vi "gRPC Status to Node Status.vi"(2 "gRPC Status":T1) -> (4 "Node Status":T10 {"Monitor Doubles"."4" format="%#_9g"; "Monitor Doubles"."3" format="%#_9g"; "Monitor Doubles"."2" format="%#_9g"; "Monitor Doubles"."1" format="%#_9g"})   [LabVIEW 2021, in "CIFCorePluginWrapper.lvlib"]
uses:
  Common/Typedef/gRPC Reported Plugin Status.ctl
  Common/Typedef/Plugin State.ctl
  Common/Typedef/Timing Statistics.ctl
  Common/Typedef/Timing Stats Base.ctl
  Common/Typedef/FIFO Statistics.ctl
  Common/Typedef/Simple Error.ctl
  Common/Typedef/Monitor Doubles.ctl
  Common/Typedef/Monitor U64.ctl
  Common/Typedef/Monitor I64.ctl
  CIFCorePlugin_client/RPC Messages/cif_plugincore_StatusData.ctl
  CIFCorePlugin_client/RPC Messages/cif_plugincore_StatusData_State.ctl
  CIFCorePlugin_client/RPC Messages/cif_plugincore_TimingStatistics.ctl
  CIFCorePlugin_client/RPC Messages/cif_plugincore_TimingStatsBasic.ctl
  CIFCorePlugin_client/RPC Messages/cif_plugincore_FifoStatistics.ctl
  CIFCorePlugin_client/RPC Messages/cif_plugincore_Error.ctl
  CIFCorePlugin_client/RPC Messages/cif_plugincore_MonitorDoubles.ctl
  CIFCorePlugin_client/RPC Messages/cif_plugincore_MonitorU64.ctl
  CIFCorePlugin_client/RPC Messages/cif_plugincore_MonitorI64.ctl
  CIFCorePluginWrapper.lvlib
  Common/CIFCoreCommon.lvlib
  CIFCorePlugin_client/CIFCorePlugin_client.lvlib
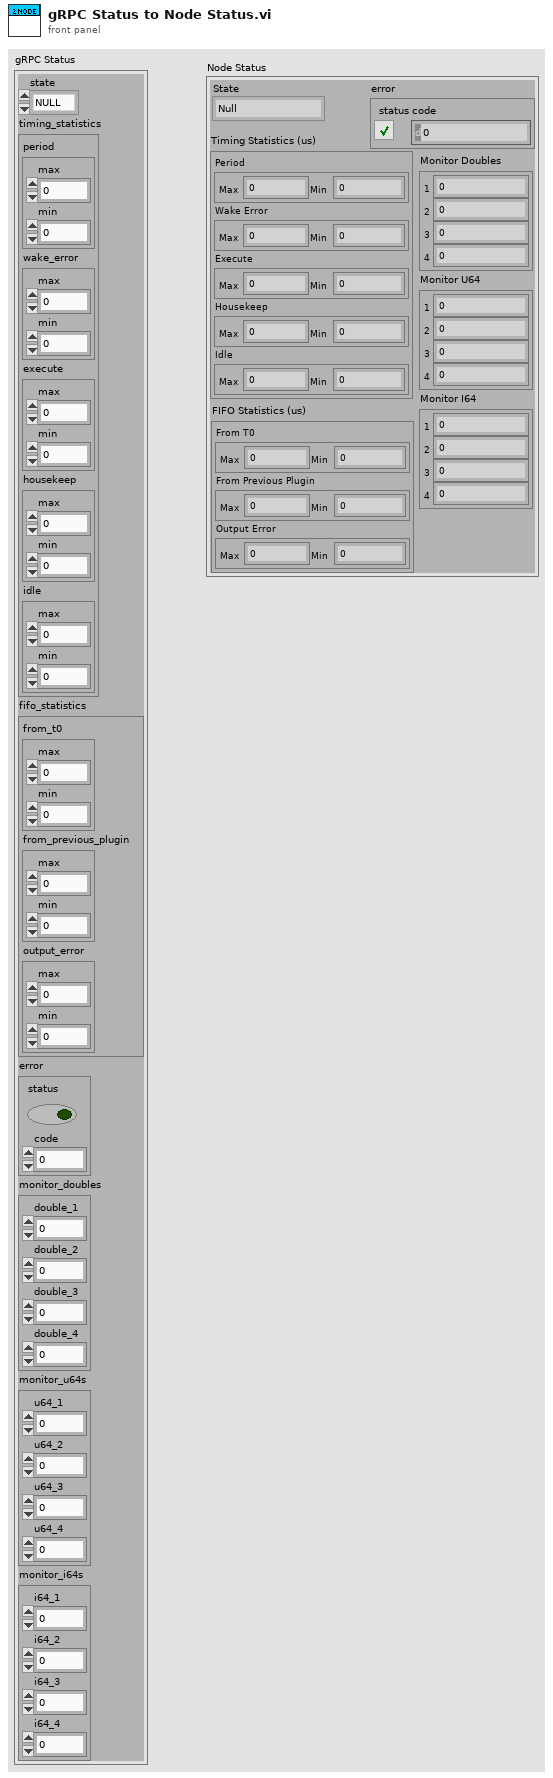
[diagram p1: front panel]
types:
  T1 = typedef "CIFCorePlugin_client.lvlib/cif_plugincore_StatusData.ctl" = cluster{"state":T2, "timing_statistics":T3, "fifo_statistics":T5, "error":T6, "monitor_doubles":T7, "monitor_u64s":T8, "monitor_i64s":T9}
  T2 = typedef "CIFCorePlugin_client.lvlib/cif_plugincore_StatusData_State.ctl" = enum32{"NULL", "CREATING", "LISTENING", "RUNNING", "CLEANINGUP", "DESTROYING"}
  T3 = typedef "CIFCorePlugin_client.lvlib/cif_plugincore_TimingStatistics.ctl" = cluster{"period":T4, "wake_error":T4, "execute":T4, "housekeep":T4, "idle":T4}
  T4 = typedef "CIFCorePlugin_client.lvlib/cif_plugincore_TimingStatsBasic.ctl" = cluster{"max":i32, "min":i32}
  T5 = typedef "CIFCorePlugin_client.lvlib/cif_plugincore_FifoStatistics.ctl" = cluster{"from_t0":T4, "from_previous_plugin":T4, "output_error":T4}
  T6 = typedef "CIFCorePlugin_client.lvlib/cif_plugincore_Error.ctl" = cluster{"status":bool, "code":i32}
  T7 = typedef "CIFCorePlugin_client.lvlib/cif_plugincore_MonitorDoubles.ctl" = cluster{"double_1":dbl, "double_2":dbl, "double_3":dbl, "double_4":dbl}
  T8 = typedef "CIFCorePlugin_client.lvlib/cif_plugincore_MonitorU64.ctl" = cluster{"u64_1":u64, "u64_2":u64, "u64_3":u64, "u64_4":u64}
  T9 = typedef "CIFCorePlugin_client.lvlib/cif_plugincore_MonitorI64.ctl" = cluster{"i64_1":i64, "i64_2":i64, "i64_3":i64, "i64_4":i64}
  T10 = typedef "CIFCoreCommon.lvlib/gRPC Reported Plugin Status.ctl" = cluster{"State":T11, "Timing Statistics (us)":T12, "FIFO Statistics (us)":T14, "error":T15, "Monitor Doubles":T16, "Monitor U64":T17, "Monitor I64":T18}
  T11 = typedef "CIFCoreCommon.lvlib/Plugin State.ctl" = enum32{"Null", "Creating", "Listening", "Running", "CleaningUp", "Destroying"}
  T12 = typedef "CIFCoreCommon.lvlib/Timing Statistics.ctl" = cluster{"Period":T13, "Wake Error":T13, "Execute":T13, "Housekeep":T13, "Idle":T13}
  T13 = typedef "CIFCoreCommon.lvlib/Timing Stats Base.ctl" = cluster{"Max":i32, "Min":i32}
  T14 = typedef "CIFCoreCommon.lvlib/FIFO Statistics.ctl" = cluster{"From T0":T13, "From Previous Plugin":T13, "Output Error":T13}
  T15 = typedef "CIFCoreCommon.lvlib/Simple Error.ctl" = cluster{"status":bool, "code":i32}
  T16 = typedef "CIFCoreCommon.lvlib/Monitor Doubles.ctl" = cluster{"1":dbl, "2":dbl, "3":dbl, "4":dbl}
  T17 = typedef "CIFCoreCommon.lvlib/Monitor U64.ctl" = cluster{"1":u64, "2":u64, "3":u64, "4":u64}
  T18 = typedef "CIFCoreCommon.lvlib/Monitor I64.ctl" = cluster{"1":i64, "2":i64, "3":i64, "4":i64}
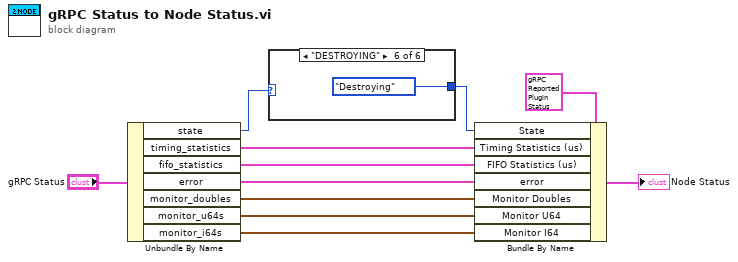
[diagram p0: block diagram]
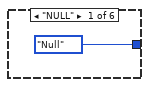
[diagram p2: hidden frame]
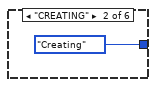
[diagram p3: hidden frame]
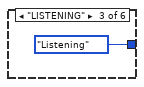
[diagram p4: hidden frame]
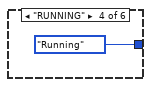
[diagram p5: hidden frame]
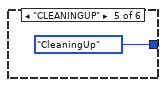
[diagram p6: hidden frame]
diagram:
  n1 = Unbundle By Name("gRPC Status") -> ("state"=w11:T2, "timing_statistics"=w10:T3, "fifo_statistics"=w9:T5, "error"=w8:T6, "monitor_doubles"=w7:T7, "monitor_u64s"=w6:T8, "monitor_i64s"=w5:T9)
  n2 = case shown="\"DESTROYING\"" w11 {
    tunnel: [Plugin_State."Null" ("State") Plugin_State."Creating" ("state") Plugin_State."Listening" ("state") Plugin_State."Running" ("state") Plugin_State."CleaningUp" ("state") Plugin_State."Destroying" ("state")] -> w3
    frame "NULL" {
    }
    frame "CREATING" {
    }
    frame "LISTENING" {
    }
    frame "RUNNING" {
    }
    frame "CLEANINGUP" {
    }
    frame "DESTROYING" {
    }
  }
  n3 = Bundle By Name(cluster=T10 {"State"=enum."Null", "Timing Statistics (us)"={"Period"={"Max"=0, "Min"=0}, "Wake Error"={"Max"=0, "Min"=0}, "Execute"={"Max"=0, "Min"=0}, "Housekeep"={"Max"=0, "Min"=0}, "Idle"={"Max"=0, "Min"=0}}, "FIFO Statistics (us)"={"From T0"={"Max"=0, "Min"=0}, "From Previous Plugin"={"Max"=0, "Min"=0}, "Output Error"={"Max"=0, "Min"=0}}, "error"={"status"=FALSE, "code"=0}, "Monitor Doubles"={"1"=0.0, "2"=0.0, "3"=0.0, "4"=0.0}, "Monitor U64"={"1"=0, "2"=0, "3"=0, "4"=0}, "Monitor I64"={"1"=0, "2"=0, "3"=0, "4"=0}} ("Node Status"), "State"=w3, "Timing Statistics (us)"=w10, "FIFO Statistics (us)"=w9, "error"=w8, "Monitor Doubles"=w7, "Monitor U64"=w6, "Monitor I64"=w5) -> (→"Node Status":T10)
